vi "Apply_Gaussian_Noise.vi"(9 "Seed in":i64, 10 "Gaussian SD in":dbl, 11 "Array in":dbl[](array[numeric])) -> (3 "Array out":dbl[](array[numeric]))   [LabVIEW 2018]
uses:
  <vilib>/Analysis/NI_AALBase.lvlib
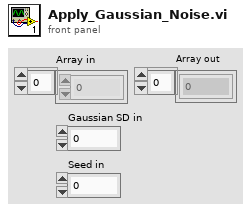
[diagram p1: front panel]
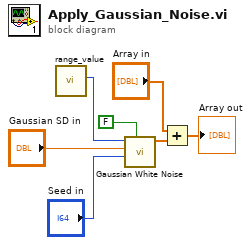
[diagram p0: block diagram]
diagram:
  n1 = call "range_value.vi"() -> ("NumBins"=w5:i32)  [unwired: 10 in, 1 out]
  n2 = call <vilib>:"Gaussian White Noise.vi"("initialize?"=FALSE, "seed"="Seed in", "standard deviation"="Gaussian SD in", "samples"=w5) -> ("Gaussian noise pattern"=w4:dbl[])  [unwired: 6 in, 1 out]
  n3 = Add(x="Array in", y=w4) -> (x+y=→"Array out":dbl[])
